vi "CRYBack To Time.vi"(9 "T(s)":dbl format="%#_6p", 10 "dt(s)":dbl=1.0 format="%#_6p", 11 "Spectrum":cdb[](array[numeric])) -> (2 "t0S":dbl format="%#_6f", 3 "timeHistory":cdb[](array[numeric]))   [LabVIEW 2013]
uses:
  <vilib>/Analysis/2dsp.llb/Inverse Complex FFT.vi
  <vilib>/Analysis/2dsp.llb/Inverse Real FFT.vi
  <vilib>/Analysis/NI_AALPro.lvlib
panel:
  out "Waveform Graph":dbl[](graph)
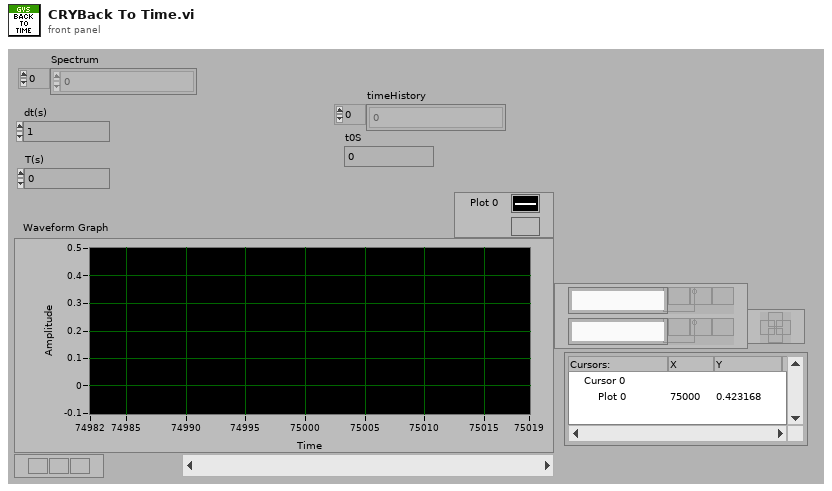
[diagram p1: front panel]
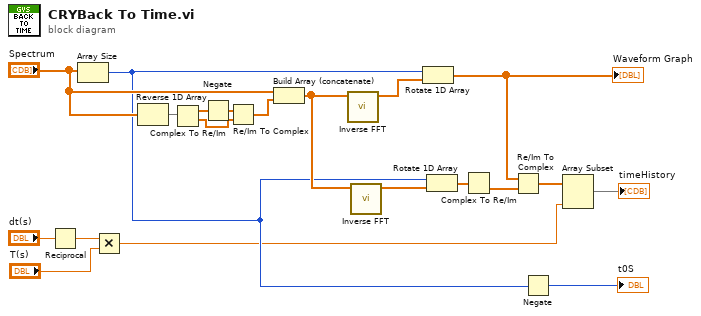
[diagram p0: block diagram]
diagram:
  n1 = Reciprocal(x="dt(s)") -> (1/x=w16:dbl)
  n2 = Array Size(array="Spectrum") -> (size(s)=w7:i32)
  n3 = Multiply(x=w16, y="T(s)") -> (x*y=w4:dbl)
  n4 = Reverse 1D Array(array="Spectrum") -> (reversed array=w13:cdb[])
  n5 = Complex To Re/Im(x + iy=w13) -> (x=w12:dbl[], y=w10:dbl[])
  n6 = Negate(x=w12) -> (-x=w11:dbl[])
  n7 = Re/Im To Complex(1:w10, 2:w11) -> (0:w9:cdb[])
  n8 = Build Array (concatenate)("Spectrum", w9) -> (w14:cdb[])
  n9 = call-poly <vilib>:"Inverse FFT.vi"("FFT {X}"=w14) -> ("X"=w19:dbl[])  [unwired: 9 in, 1 out]
  n10 = call-poly <vilib>:"Inverse FFT.vi"("FFT {X}"=w14) -> ("X"=w18:cdb[])  [unwired: 9 in, 1 out]
  n11 = Rotate 1D Array(1:w19, 2:w7) -> (0:w5:dbl[])
  "Waveform Graph" <- w5
  n12 = Rotate 1D Array(1:w18, 2:w7) -> (0:w8:cdb[])
  n13 = Complex To Re/Im(x + iy=w8) -> (y=w3:dbl[])  [unwired: 1 out]
  n14 = Re/Im To Complex(1:w3, 2:w5) -> (0:w2:cdb[])
  n15 = Negate(x=w7) -> (-x=→"t0S":i32)
  n16 = Array Subset(array=w2, length=w4) -> (→"timeHistory":cdb[])  [unwired: 1 in]
